vi "Find Most Recent File.vi"(8 "error in (no error)":errorcluster, 11 "All Files in Dir":path[](array[path])) -> (0 "error out":errorcluster, 3 "Path":path)   [LabVIEW 2019, in "Build.lvlib"]
uses:
  Build.lvlib
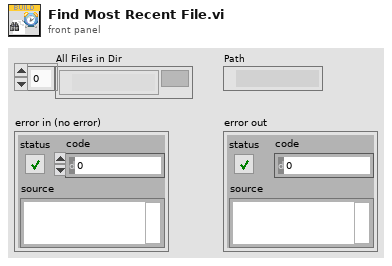
[diagram p1: front panel]
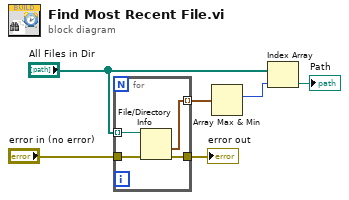
[diagram p0: block diagram]
diagram:
  n1 = for {
    tunnel: "All Files in Dir" -> [w10] mode=indexing
    tunnel: [w9] -> w1 mode=indexing
    tunnel: "error in (no error)" -> [w8]
    tunnel: [w7] -> w6
    n2 = File/Directory Info(path=w10, error in=w8) -> (last mod=w9:timestamp, error out=w7:errorcluster)  [unwired: 5 out]
  }
  "error out" <- w6
  n3 = Array Max & Min(array=w1) -> (max index (indices)=w2:i32)  [unwired: 3 out]
  n4 = Index Array(array="All Files in Dir", index=w2) -> (element=→"Path":path)
